vi "arduinoOpenValveAnsSolenoidsMs.vi"() -> ()   [LabVIEW 2012]
uses:
  GlobalValves.vi
panel:
  in  "milliseconds to wait after solenoid\nrelease":u32=100
  in  "valve data close":bool[](array[boolean])=[FALSE, FALSE, FALSE, FALSE, FALSE, FALSE, FALSE, FALSE]
  in  "valve data release solenoid":bool[](array[boolean])=[FALSE, FALSE, FALSE, FALSE, FALSE, FALSE, FALSE, FALSE]
  in  "milliseconds to wait":u32=100
  in  "valve data open":bool[](array[boolean])=[TRUE, FALSE, FALSE, FALSE, FALSE, FALSE, FALSE, FALSE]
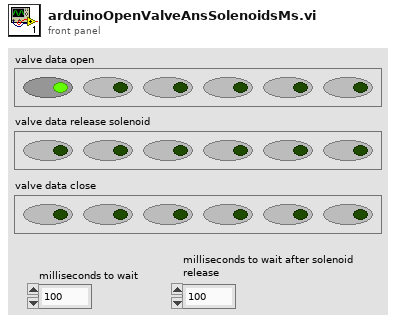
[diagram p1: front panel]
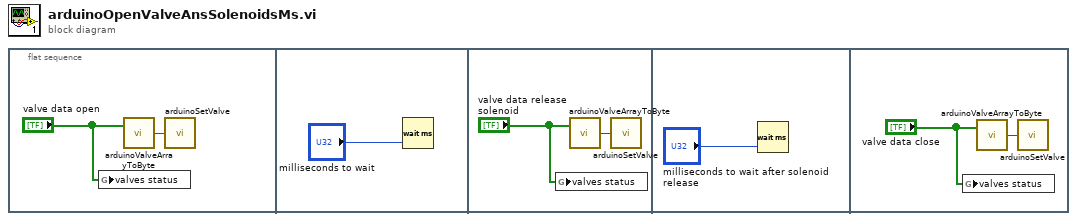
[diagram p0: block diagram]
diagram:
  n1 = flat-sequence {
    frame #0 {
      n2 = global write "GlobalValves.vi" "valves status"("valve data open") -> ()
      n3 = call "arduinoValveArrayToByte.vi"("valve data open"="valve data open") -> ("output"=w2:u8)  [unwired: 1 in]
      n4 = call "arduinoSetValve.vi"("command"=w2) -> ()
    }
    frame #1 {
      n5 = Wait (ms)(milliseconds to wait="milliseconds to wait") -> ()  [unwired: 1 out]
    }
    frame #2 {
      n6 = global write "GlobalValves.vi" "valves status"("valve data release solenoid") -> ()
      n7 = call "arduinoValveArrayToByte.vi"("valve data open"="valve data release solenoid") -> ("output"=w5:u8)  [unwired: 1 in]
      n8 = call "arduinoSetValve.vi"("command"=w5) -> ()
    }
    frame #3 {
      n9 = Wait (ms)(milliseconds to wait="milliseconds to wait after solenoid\nrelease") -> ()  [unwired: 1 out]
    }
    frame #4 {
      n10 = global write "GlobalValves.vi" "valves status"("valve data close") -> ()
      n11 = call "arduinoValveArrayToByte.vi"("valve data open"="valve data close") -> ("output"=w8:u8)  [unwired: 1 in]
      n12 = call "arduinoSetValve.vi"("command"=w8) -> ()
    }
  }
